vi "Error Cluster From Error Code (G8).vi"(4 "is warning? (False)":bool, 5 "show call chain? (False)":bool, 6 "error in (no error)":errorcluster, 8 "error message (\"\")":string, 9 "error code (0)":i32) -> (0 "error out":errorcluster)   [LabVIEW 2014, in "Utilities.lvlib"]
doc: "Converts an error or warning code to an error cluster. This VI is useful when you receive a return value from a DLL call or when you return user-defined error codes."
uses:
  <vilib>/Utility/error.llb/whitespace.ctl
  Utilities.lvlib
panel:
  in  "call chain header":string="\n<b>Complete call chain:</b>"
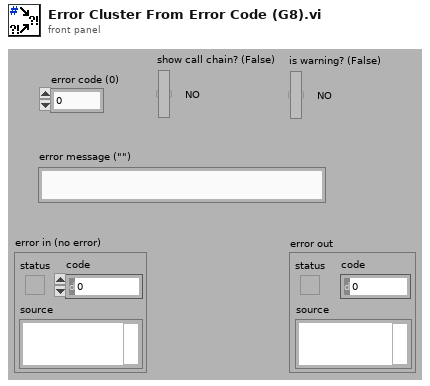
[diagram p1: front panel]
types:
  T1 = typedef "whitespace.ctl" = u16
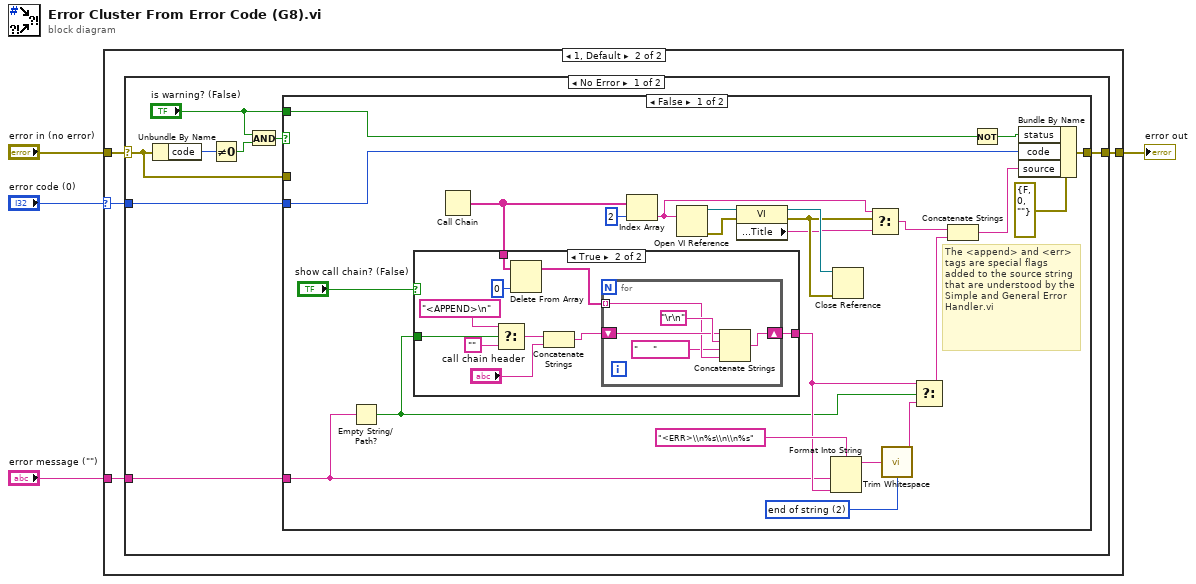
[diagram p0: block diagram]
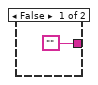
[diagram p3: hidden frame]
diagram:
  n1 = case shown="1, Default" "error code (0)" {
    selector: "error code (0)" -> [_ w7]
    tunnel: [w5 w9] -> w4
    tunnel: "error in (no error)" -> [w5 w8]
    tunnel: "error message (\"\")" -> [_ w6]
    frame 0 {
      # "If the error code in equals zero, then propagate the error in cluster regardless of its value."
    }
    frame 1, Default {
      n2 = case shown="No Error" w8 {
        selector: w8 -> [w12 w59]
        tunnel: [w17 w59] -> w9
        tunnel: w7 -> [w16 _]
        tunnel: w6 -> [w10 _]
        frame No Error {
          n3 = Unbundle By Name(w12) -> ("code"=w15:i32)
          n4 = Not Equal To 0?(x=w15) -> (x != 0?=w13:bool)
          n5 = And(x="is warning? (False)", y=w13) -> (x .and. y?=w14:bool)
          n6 = case shown="False" w14 {
            tunnel: [w41 w58] -> w17
            tunnel: w16 -> [w37 _]
            tunnel: w12 -> [_ w58]
            tunnel: "is warning? (False)" -> [w27 _]
            tunnel: w10 -> [w22 _]
            frame False {
              w18 = T1 2 items=["both", "start of string", "end of string"] ("location (both)")
              # "The <append> and <err> tags are special flags added to the source string that are understood by the Simple and General Error Handler.vi"
              n7 = Empty String/Path?(string/path=w22) -> (empty?=w21:bool)
              n8 = Call Chain() -> (call chain=w32:string[])
              n9 = case shown="True" "show call chain? (False)" {
                tunnel: ["" w52] -> w24
                tunnel: w32 -> [_ w50]
                tunnel: w21 -> [_ w46]
                frame False {
                }
                frame True {
                  n10 = Select(t="<APPEND>\n", s=w46, f="") -> (s? t:f=w43:string)
                  n11 = Delete From Array(array=w50, index=0) -> (array with subset deleted=w49:string[])  [unwired: 1 in, 1 out]
                  n12 = Concatenate Strings(w43, "call chain header") -> (w47:string)
                  n13 = for {
                    tunnel: w49 -> [w54] mode=indexing
                    shift-right: [w57] -> w52
                    shift-left: w47 -> [w55]
                    n14 = Concatenate Strings(w55, "\r\n", "     ", w54) -> (w57:string)
                  }
                }
              }
              n15 = Index Array(array=w32, index=2) -> (element=w30:string)
              n16 = Open VI Reference(vi path=w30) -> (vi reference=w35:refnum<vi>, error out=w34:errorcluster)  [unwired: 5 in]
              n17 = property class="VI"(reference=w35, error in=w34) -> (reference out=w33:refnum<vi>, error out=w31:errorcluster, "Front Panel Window:Title"=w29:string)
              n18 = Format Into String(format string="<ERR>\\n%s\\n\\n%s", w22, w24) -> (resulting string=w20:string)  [unwired: 2 in, 1 out]
              n19 = Close Reference(reference=w33, error in (no error)=w31) -> ()  [unwired: 1 out]
              n20 = Select(t=w30, s=w31, f=w29) -> (s? t:f=w28:string)
              n21 = call <vilib>:"Trim Whitespace.vi"("string"=w20, "location (both)"=w18) -> ("trimmed string"=w19:string)
              n22 = Select(t=w24, s=w21, f=w19) -> (s? t:f=w23:string)
              n23 = Concatenate Strings(w28, w23) -> (w39:string)
              n24 = Not(x=w27) -> (.not. x?=w38:bool)
              n25 = Bundle By Name(cluster=errorcluster {"status"=FALSE, "code"=0, "source"=""} ("error out"), "status"=w38, "code"=w37, "source"=w39) -> (w41:errorcluster)
            }
            frame True {
              # "If the error code input is setting a warning, and a warning is already set on the wire, then we\ngo with the one already on the wire."
            }
          }
        }
        frame Error {
          # "An error in trumps any error code input."
        }
      }
    }
  }
  "error out" <- w4
